vi "deinitialize.vi"(0 "HGF_DSCMonitor":refnum<class "HGF_DSCMonitor.lvclass">, 5 "error in (no error)":errorcluster) -> (19 "error out":errorcluster)   [LabVIEW 2012, in "HGF_DSC.lvlib" / "HGF_DSCMonitor.lvclass"]
doc: "This is a dynamic dispatch VI. It can be overwritten by childclasses to release allocated recources."
uses:
  HGF_DSCMonitor.lvclass
  HGF_SV/HGF_Monitor/HGF_Monitor.lvclass
  HGF_DSCMonitor.lvclass/HGF_DSCMonitor.ctl
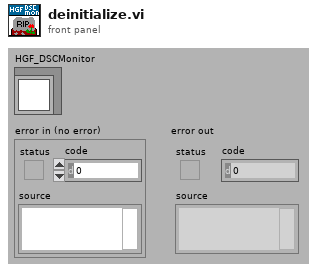
[diagram p1: front panel]
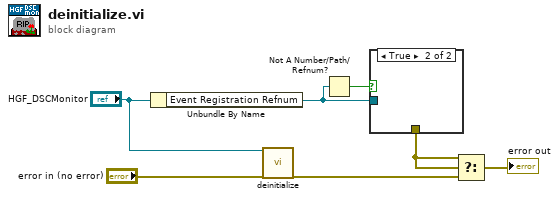
[diagram p0: block diagram]
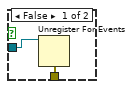
[diagram p2: hidden frame]
diagram:
  n1 = Unbundle By Name("HGF_DSCMonitor") -> ("Event Registration Refnum"=w3:refnum<event-registration>)
  n2 = call-parent "deinitialize.vi"("HGF_Factory"="HGF_DSCMonitor", "error in (no error)"="error in (no error)") -> ("error out"=w5:errorcluster)  [unwired: 17 out]
  n3 = Not A Number/Path/Refnum?(number/path/refnum=w3) -> (NaN/Path/Refnum?=w2:bool)
  n4 = case shown="True" w2 {
    tunnel: [w9 _] -> w1
    tunnel: w3 -> [w8 _]
    frame False {
      n5 = Unregister For Events(event registration refnum=w8) -> (error out=w9:errorcluster)  [unwired: 1 in]
    }
    frame True {
    }
  }
  n6 = Select(t=w1, s=w1, f=w5) -> (s? t:f=→"error out":errorcluster)
